vi "PolXYGraph.vi"(0 "Interpreted Values":sgl[](array[numeric]) format="%.2f", 3 "x-indexes":i32[](array[numeric]), 5 "y-indexes":i32[](array[numeric])) -> (7 "XY Graph":cluster{sgl, sgl}[](graph))   [LabVIEW 2012]
doc: "Indexes the interpreted values at the given locations and outputs a number of points to display on an XY Graphs"
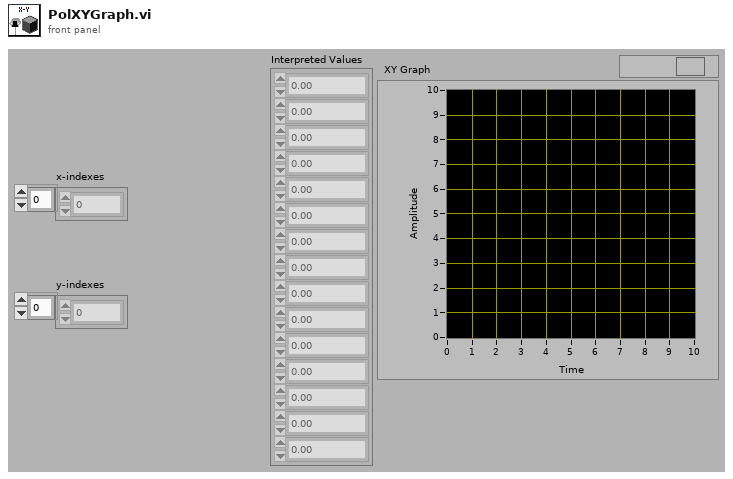
[diagram p1: front panel]
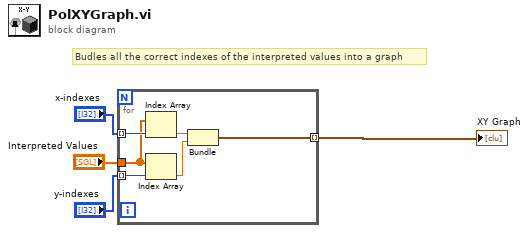
[diagram p0: block diagram]
diagram:
  # "Budles all the correct indexes of the interpreted values into a graph"
  n1 = for {
    tunnel: "Interpreted Values" -> [w9]
    tunnel: "x-indexes" -> [w10] mode=indexing
    tunnel: "y-indexes" -> [w8] mode=indexing
    tunnel: [w5] -> w1 mode=indexing
    n2 = Index Array(array=w9, index=w10) -> (element=w7:sgl)
    n3 = Index Array(array=w9, index=w8) -> (element=w6:sgl)
    n4 = Bundle(w7, w6) -> (w5:cluster{sgl, sgl})  [unwired: 1 in]
  }
  "XY Graph" <- w1
